vi "Normalize and Dark Correct.vi"(8 "Dark Int Time":dbl format="%#_13g", 9 "Dark Counts":dbl[](array[numeric]), 10 "Measured Int Time":dbl format="%#_13g", 11 "Measured Counts":dbl[](array[numeric])) -> (3 "Normalized and Dark Corrected":dbl[](array[numeric]))   [LabVIEW 2013, in "AvaSpec.lvlib"]
uses:
  AvaSpec.lvlib
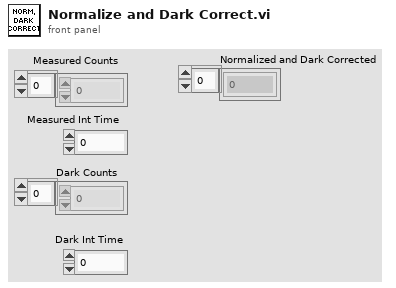
[diagram p1: front panel]
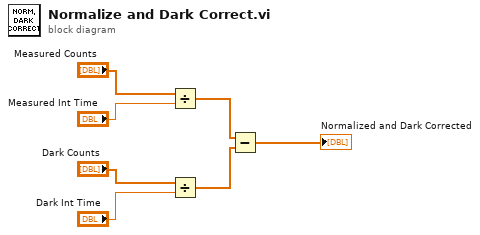
[diagram p0: block diagram]
diagram:
  n1 = Divide(x="Measured Counts", y="Measured Int Time") -> (x/y=w3:dbl[])
  n2 = Divide(x="Dark Counts", y="Dark Int Time") -> (x/y=w2:dbl[])
  n3 = Subtract(x=w3, y=w2) -> (x-y=→"Normalized and Dark Corrected":dbl[])
